vi "Test TS530A Remote Control.vi"() -> ()   [LabVIEW 2012]
doc: "Application example"
uses:
  <vilib>/Analysis/baseanly.llb/Mean (DBL).vi
  <vilib>/Analysis/NI_AALBase.lvlib
panel:
  out "SET POINT":u16
  out "MEASURED":dbl
  out "RESULTS":dbl[](array[numeric])
  in  "WHAT TO TEST":enum16{"PARAMS AND SET POINT", "ONLY SET POINT"}(ring)=enum."ONLY SET POINT"
  in  "VISA RESOURCE":refnum<visa-resource-name>="COM4"
  # "Test TS530A Remote Control.vi"
  # "NOTE: The 37-way data cable connecting the AVS-47B and TS-530A is needed for this test\n\nThis test VI goes through all PID parameters, turning on each of the TS-530A front panel\nstatus LEDs if the \"what to test\" control is \"params and set point\".  Then the VI \nproceeds to program the analog set point to values 2^n where n=0...14. The \"measured\" \nindicator shows the last result, while the \"results\" array is filled after the VI has run\nto the end. \n\nThe measured set point values may deviate from the ideal values by some hundred\nmicrovolts because of the finite accuracy of the D/A and A/D converters. \n    Operating range of the D/A converter starts from 1 and therefore the  very lowest \nreadings (<10..30) may be quite erroneous."
  # "1"
  # "2"
  # "4"
  # "8"
  # "16"
  # "32"
  # "64"
  # "128"
  # "256"
  # "512"
  # "1024"
  # "2048"
  # "4096"
  # "8192"
  # "16384"
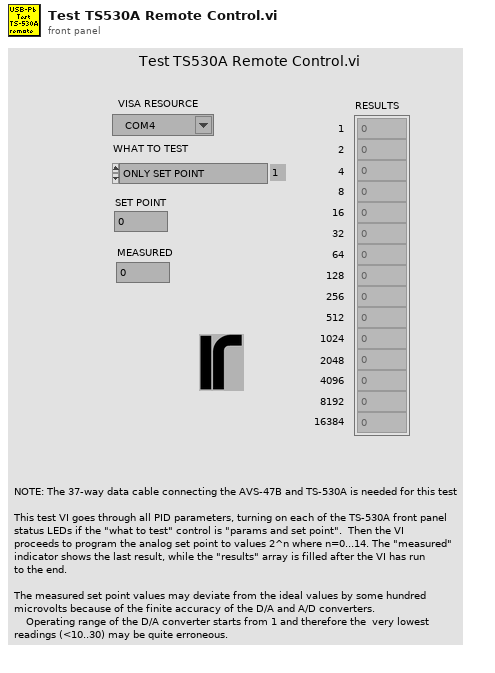
[diagram p1: front panel]
types:
  T1 = cluster{"VISA RESOURCE":refnum<visa-resource-name>, "PICOBUS ADDRESS":u8, "DISABLE AL":u8, "REMOTE":u8, "INPUT":u8, "CHANNEL":u8, "RANGE":u8, "EXCITATION":u8, "DISPLAY":u8, "DIGITAL REFERENCE":u16, "SET POINT":dbl, "PROP GAIN":u8, "INTG":u8, "DERIV":u8, "POWER BIAS":u8, "POWER RANGE":u8, "INFO STRING":string, "HEATER RESISTANCE":dbl, "INTERVAL":u8, " SENSOR dR/dT":u8}
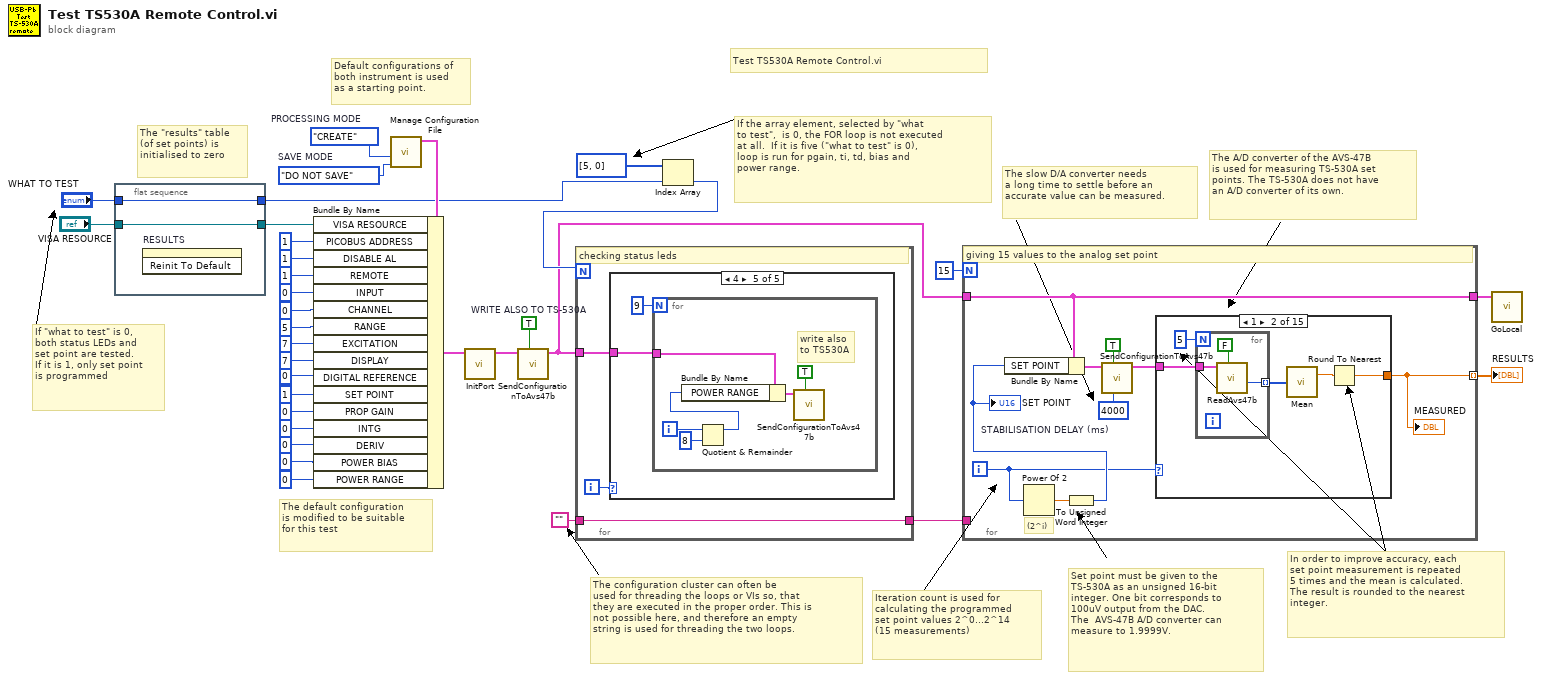
[diagram p0: block diagram]
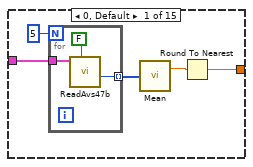
[diagram p2: hidden frame]
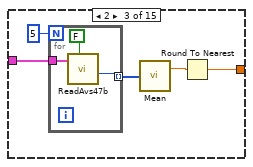
[diagram p3: hidden frame]
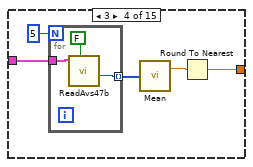
[diagram p4: hidden frame]
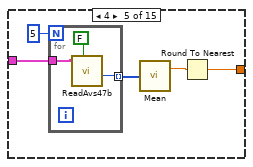
[diagram p5: hidden frame]
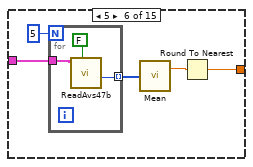
[diagram p6: hidden frame]
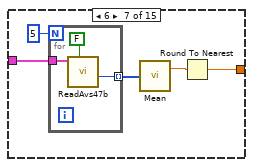
[diagram p7: hidden frame]
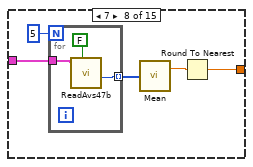
[diagram p8: hidden frame]
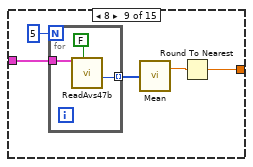
[diagram p9: hidden frame]
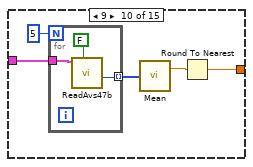
[diagram p10: hidden frame]
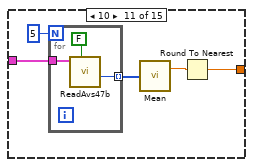
[diagram p11: hidden frame]
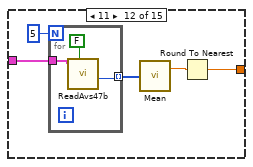
[diagram p12: hidden frame]
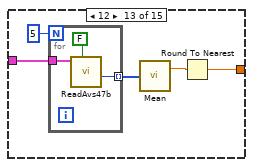
[diagram p13: hidden frame]
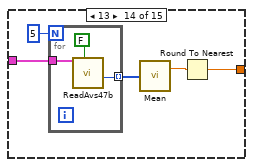
[diagram p14: hidden frame]
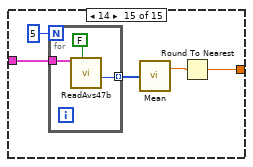
[diagram p15: hidden frame]
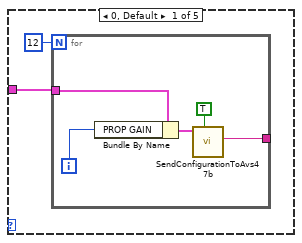
[diagram p16: hidden frame]
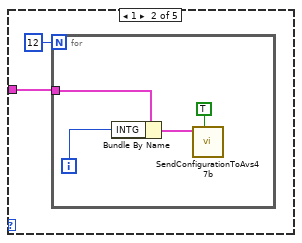
[diagram p17: hidden frame]
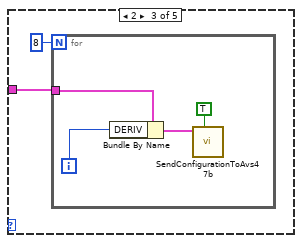
[diagram p18: hidden frame]
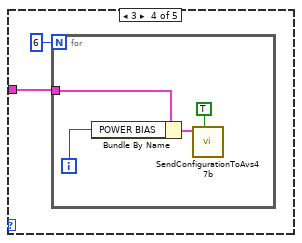
[diagram p19: hidden frame]
diagram:
  w3 = enum16{"DO NOT SAVE", "SAVE .CNF FILE"}."DO NOT SAVE"  # SAVE MODE
  w4 = enum16{"NONE", "READ", "CREATE"}."CREATE"  # PROCESSING MODE
  w17 = TRUE  # WRITE ALSO TO TS-530A
  # "Default configurations of \nboth instrument is used\nas a starting point."
  # "Test TS530A Remote Control.vi"
  # "The A/D converter of the AVS-47B\nis used for measuring TS-530A set\npoints. The TS-530A does not have\nan A/D converter of its own."
  # "If the array element, selected by \"what\nto test\",  is 0, the FOR loop is not executed \nat all.  If it is five (\"what to test\" is 0),\nloop is run for pgain, ti, td, bias and \npower range."
  # "The configuration cluster can often be\nused for threading the loops or VIs so, that \nthey are executed in the proper order. This is \nnot possible here, and therefore an empty \nstring is used for threading the two loops."
  # "Iteration count is used for\ncalculating the programmed\nset point values 2^0...2^14\n(15 measurements)"
  # "In order to improve accuracy, each \nset point measurement is repeated \n5 times and the mean is calculated. \nThe result is rounded to the nearest \ninteger."
  # "The slow D/A converter needs\na long time to settle before an\naccurate value can be measured."
  # "Set point must be given to the \nTS-530A as an unsigned 16-bit \ninteger. One bit corresponds to\n100uV output from the DAC. \nThe  AVS-47B A/D converter can \nmeasure to 1.9999V."
  # "If \"what to test\" is 0,\nboth status LEDs and \nset point are tested.\nIf it is 1, only set point\nis programmed"
  # "The default configuration\nis modified to be suitable\nfor this test"
  # "The \"results\" table\n(of set points) is \ninitialised to zero"
  n1 = flat-sequence {
    tunnel: "VISA RESOURCE" -> [w35]
    tunnel: [w35] -> w11
    tunnel: "WHAT TO TEST" -> [w34]
    tunnel: [w34] -> w9
    frame #0 {
      n2 = invoke on="RESULTS" class="Arr (strict)" method="Reinit To Default"() -> ()  [unwired: 3 in, 3 out]
    }
  }
  n3 = call "Manage Configuration File.vi"("SAVE MODE"=w3, "PROCESSING MODE"=w4) -> ("CONFIGURATION CLUSTER OUT"=w33:T1)  [unwired: 9 in]
  n4 = Bundle By Name(cluster=w33, "VISA RESOURCE"=w11, "PICOBUS ADDRESS"=u8 1, "DISABLE AL"=u8 1 ("PICOBUS ADDRESS"), "REMOTE"=u8 1 ("PICOBUS ADDRESS"), "INPUT"=u8 0 ("PICOBUS ADDRESS"), "CHANNEL"=u8 0 ("PICOBUS ADDRESS"), "RANGE"=u8 5 ("PICOBUS ADDRESS"), "EXCITATION"=u8 7 ("PICOBUS ADDRESS"), "DISPLAY"=u8 7 ("PICOBUS ADDRESS"), "DIGITAL REFERENCE"=u16 0, "SET POINT"=u16 1, "PROP GAIN"=u8 0 ("PICOBUS ADDRESS"), "INTG"=u8 0 ("PICOBUS ADDRESS"), "DERIV"=u8 0 ("PICOBUS ADDRESS"), "POWER BIAS"=u8 0 ("PICOBUS ADDRESS"), "POWER RANGE"=u8 0 ("PICOBUS ADDRESS")) -> (w2:T1)
  n5 = call "InitPort.vi"("CONFIGURATION CLUSTER"=w2) -> ("UNMODIFIED CONFIGURATION CLUSTER"=w1:T1)  [unwired: 6 in, 2 out]
  n6 = call "SendConfigurationToAvs47b.vi"("WRITE ALSO TO TS-530A"=w17, "CONFIGURATION CLUSTER"=w1) -> ("UNMODIFIED CONFIGURATION CLUSTER"=w7:T1)  [unwired: 6 in, 3 out]
  n7 = Index Array(array=i32[] [5, 0], index=w9) -> (element=w13:i32)
  n8 = for {
    N: w13 -> [_]
    tunnel: w7 -> [w37]
    tunnel: "" -> [w36]
    tunnel: [w36] -> w5
    i -> [w38]
    # "checking status leds"
    n9 = case shown="4" w38 {
      tunnel: w37 -> [w39 w46 w52 w58 w64]
      frame 0, Default {
        n10 = for {
          N: 12 -> [_]
          tunnel: w39 -> [w42]
          tunnel: [w41] -> _
          i -> [w45]
          n11 = Bundle By Name(cluster=w42, "PROP GAIN"=w45) -> (w44:T1)
          n12 = call "SendConfigurationToAvs47b.vi"("WRITE ALSO TO TS-530A"=TRUE, "CONFIGURATION CLUSTER"=w44) -> ("AVS47B TXSTR"=w41:string)  [unwired: 6 in, 3 out]
        }
      }
      frame 1 {
        n13 = for {
          N: 12 -> [_]
          tunnel: w46 -> [w48]
          i -> [w51]
          n14 = Bundle By Name(cluster=w48, "INTG"=w51) -> (w50:T1)
          n15 = call "SendConfigurationToAvs47b.vi"("WRITE ALSO TO TS-530A"=TRUE, "CONFIGURATION CLUSTER"=w50) -> ()  [unwired: 6 in, 4 out]
        }
      }
      frame 2 {
        n16 = for {
          N: 8 -> [_]
          tunnel: w52 -> [w54]
          i -> [w57]
          n17 = Bundle By Name(cluster=w54, "DERIV"=w57) -> (w56:T1)
          n18 = call "SendConfigurationToAvs47b.vi"("WRITE ALSO TO TS-530A"=TRUE, "CONFIGURATION CLUSTER"=w56) -> ()  [unwired: 6 in, 4 out]
        }
      }
      frame 3 {
        n19 = for {
          N: 6 -> [_]
          tunnel: w58 -> [w60]
          i -> [w63]
          n20 = Bundle By Name(cluster=w60, "POWER BIAS"=w63) -> (w62:T1)
          n21 = call "SendConfigurationToAvs47b.vi"("WRITE ALSO TO TS-530A"=TRUE, "CONFIGURATION CLUSTER"=w62) -> ()  [unwired: 6 in, 4 out]
        }
      }
      frame 4 {
        n22 = for {
          N: 9 -> [_]
          tunnel: w64 -> [w66]
          i -> [w69]
          # "write also \nto TS530A"
          n23 = Quotient & Remainder(x=w69, y=8) -> (x-y*floor(x/y)=w67:i32)  [unwired: 1 out]
          n24 = Bundle By Name(cluster=w66, "POWER RANGE"=w67) -> (w71:T1)
          n25 = call "SendConfigurationToAvs47b.vi"("WRITE ALSO TO TS-530A"=TRUE, "CONFIGURATION CLUSTER"=w71) -> ()  [unwired: 6 in, 4 out]
        }
      }
    }
  }
  n26 = for {
    N: 15 -> [_]
    tunnel: w7 -> [w73]
    tunnel: [w73] -> w15
    tunnel: [w72] -> w8 mode=indexing
    tunnel: w5 -> [_]
    i -> [w75]
    w76 = 4000  # STABILISATION DELAY (ms)
    # "(2^i)"
    # "giving 15 values to the analog set point"
    n27 = Power Of 2(x=w75) -> (2^x=w78:dbl)
    n28 = To Unsigned Word Integer(number=w78) -> (unsigned 16bit integer=w77:u16)
    "SET POINT" <- w77
    n29 = Bundle By Name(cluster=w73, "SET POINT"=w77) -> (w80:T1)
    n30 = call "SendConfigurationToAvs47b.vi"("STABILISATION DELAY (ms)"=w76, "WRITE ALSO TO TS-530A"=TRUE, "CONFIGURATION CLUSTER"=w80) -> ("UNMODIFIED CONFIGURATION CLUSTER"=w74:T1)  [unwired: 5 in, 3 out]
    n31 = case shown="1" w75 {
      tunnel: w74 -> [w85 w93 w101 w109 w117 w125 w133 w141 w149 w157 w165 w173 w181 w189 w197]
      tunnel: [w81 w89 w97 w105 w113 w121 w129 w137 w145 w153 w161 w169 w177 w185 w193] -> w72
      frame 0, Default {
        n32 = for {
          N: 5 -> [_]
          tunnel: w85 -> [w88]
          tunnel: [w87] -> w83 mode=indexing
          n33 = call "ReadAvs47b.vi"("SYNCHRONISE TO ADC"=FALSE ("SYNCHRONIZE TO ADC"), "CONFIGURATION CLUSTER"=w88) -> ("ADC"=w87:i32)  [unwired: 4 in, 5 out]
        }
        n34 = call-poly <vilib>:"Mean.vi"("X"=w83) -> ("mean"=w82:dbl)  [unwired: 1 out]
        n35 = Round To Nearest(number=w82) -> (nearest integer value=w81:dbl)
      }
      frame 1 {
        n36 = for {
          N: 5 -> [_]
          tunnel: w93 -> [w96]
          tunnel: [w95] -> w91 mode=indexing
          n37 = call "ReadAvs47b.vi"("SYNCHRONISE TO ADC"=FALSE ("SYNCHRONIZE TO ADC"), "CONFIGURATION CLUSTER"=w96) -> ("ADC"=w95:i32)  [unwired: 4 in, 5 out]
        }
        n38 = call-poly <vilib>:"Mean.vi"("X"=w91) -> ("mean"=w90:dbl)  [unwired: 1 out]
        n39 = Round To Nearest(number=w90) -> (nearest integer value=w89:dbl)
      }
      frame 2 {
        n40 = for {
          N: 5 -> [_]
          tunnel: w101 -> [w103]
          tunnel: [w102] -> w99 mode=indexing
          n41 = call "ReadAvs47b.vi"("SYNCHRONISE TO ADC"=FALSE ("SYNCHRONIZE TO ADC"), "CONFIGURATION CLUSTER"=w103) -> ("ADC"=w102:i32)  [unwired: 4 in, 5 out]
        }
        n42 = call-poly <vilib>:"Mean.vi"("X"=w99) -> ("mean"=w98:dbl)  [unwired: 1 out]
        n43 = Round To Nearest(number=w98) -> (nearest integer value=w97:dbl)
      }
      frame 3 {
        n44 = for {
          N: 5 -> [_]
          tunnel: w109 -> [w111]
          tunnel: [w110] -> w107 mode=indexing
          n45 = call "ReadAvs47b.vi"("SYNCHRONISE TO ADC"=FALSE ("SYNCHRONIZE TO ADC"), "CONFIGURATION CLUSTER"=w111) -> ("ADC"=w110:i32)  [unwired: 4 in, 5 out]
        }
        n46 = call-poly <vilib>:"Mean.vi"("X"=w107) -> ("mean"=w106:dbl)  [unwired: 1 out]
        n47 = Round To Nearest(number=w106) -> (nearest integer value=w105:dbl)
      }
      frame 4 {
        n48 = for {
          N: 5 -> [_]
          tunnel: w117 -> [w119]
          tunnel: [w118] -> w115 mode=indexing
          n49 = call "ReadAvs47b.vi"("SYNCHRONISE TO ADC"=FALSE ("SYNCHRONIZE TO ADC"), "CONFIGURATION CLUSTER"=w119) -> ("ADC"=w118:i32)  [unwired: 4 in, 5 out]
        }
        n50 = call-poly <vilib>:"Mean.vi"("X"=w115) -> ("mean"=w114:dbl)  [unwired: 1 out]
        n51 = Round To Nearest(number=w114) -> (nearest integer value=w113:dbl)
      }
      frame 5 {
        n52 = for {
          N: 5 -> [_]
          tunnel: w125 -> [w127]
          tunnel: [w126] -> w123 mode=indexing
          n53 = call "ReadAvs47b.vi"("SYNCHRONISE TO ADC"=FALSE ("SYNCHRONIZE TO ADC"), "CONFIGURATION CLUSTER"=w127) -> ("ADC"=w126:i32)  [unwired: 4 in, 5 out]
        }
        n54 = call-poly <vilib>:"Mean.vi"("X"=w123) -> ("mean"=w122:dbl)  [unwired: 1 out]
        n55 = Round To Nearest(number=w122) -> (nearest integer value=w121:dbl)
      }
      frame 6 {
        n56 = for {
          N: 5 -> [_]
          tunnel: w133 -> [w135]
          tunnel: [w134] -> w131 mode=indexing
          n57 = call "ReadAvs47b.vi"("SYNCHRONISE TO ADC"=FALSE ("SYNCHRONIZE TO ADC"), "CONFIGURATION CLUSTER"=w135) -> ("ADC"=w134:i32)  [unwired: 4 in, 5 out]
        }
        n58 = call-poly <vilib>:"Mean.vi"("X"=w131) -> ("mean"=w130:dbl)  [unwired: 1 out]
        n59 = Round To Nearest(number=w130) -> (nearest integer value=w129:dbl)
      }
      frame 7 {
        n60 = for {
          N: 5 -> [_]
          tunnel: w141 -> [w143]
          tunnel: [w142] -> w139 mode=indexing
          n61 = call "ReadAvs47b.vi"("SYNCHRONISE TO ADC"=FALSE ("SYNCHRONIZE TO ADC"), "CONFIGURATION CLUSTER"=w143) -> ("ADC"=w142:i32)  [unwired: 4 in, 5 out]
        }
        n62 = call-poly <vilib>:"Mean.vi"("X"=w139) -> ("mean"=w138:dbl)  [unwired: 1 out]
        n63 = Round To Nearest(number=w138) -> (nearest integer value=w137:dbl)
      }
      frame 8 {
        n64 = for {
          N: 5 -> [_]
          tunnel: w149 -> [w151]
          tunnel: [w150] -> w147 mode=indexing
          n65 = call "ReadAvs47b.vi"("SYNCHRONISE TO ADC"=FALSE ("SYNCHRONIZE TO ADC"), "CONFIGURATION CLUSTER"=w151) -> ("ADC"=w150:i32)  [unwired: 4 in, 5 out]
        }
        n66 = call-poly <vilib>:"Mean.vi"("X"=w147) -> ("mean"=w146:dbl)  [unwired: 1 out]
        n67 = Round To Nearest(number=w146) -> (nearest integer value=w145:dbl)
      }
      frame 9 {
        n68 = for {
          N: 5 -> [_]
          tunnel: w157 -> [w159]
          tunnel: [w158] -> w155 mode=indexing
          n69 = call "ReadAvs47b.vi"("SYNCHRONISE TO ADC"=FALSE ("SYNCHRONIZE TO ADC"), "CONFIGURATION CLUSTER"=w159) -> ("ADC"=w158:i32)  [unwired: 4 in, 5 out]
        }
        n70 = call-poly <vilib>:"Mean.vi"("X"=w155) -> ("mean"=w154:dbl)  [unwired: 1 out]
        n71 = Round To Nearest(number=w154) -> (nearest integer value=w153:dbl)
      }
      frame 10 {
        n72 = for {
          N: 5 -> [_]
          tunnel: w165 -> [w167]
          tunnel: [w166] -> w163 mode=indexing
          n73 = call "ReadAvs47b.vi"("SYNCHRONISE TO ADC"=FALSE ("SYNCHRONIZE TO ADC"), "CONFIGURATION CLUSTER"=w167) -> ("ADC"=w166:i32)  [unwired: 4 in, 5 out]
        }
        n74 = call-poly <vilib>:"Mean.vi"("X"=w163) -> ("mean"=w162:dbl)  [unwired: 1 out]
        n75 = Round To Nearest(number=w162) -> (nearest integer value=w161:dbl)
      }
      frame 11 {
        n76 = for {
          N: 5 -> [_]
          tunnel: w173 -> [w175]
          tunnel: [w174] -> w171 mode=indexing
          n77 = call "ReadAvs47b.vi"("SYNCHRONISE TO ADC"=FALSE ("SYNCHRONIZE TO ADC"), "CONFIGURATION CLUSTER"=w175) -> ("ADC"=w174:i32)  [unwired: 4 in, 5 out]
        }
        n78 = call-poly <vilib>:"Mean.vi"("X"=w171) -> ("mean"=w170:dbl)  [unwired: 1 out]
        n79 = Round To Nearest(number=w170) -> (nearest integer value=w169:dbl)
      }
      frame 12 {
        n80 = for {
          N: 5 -> [_]
          tunnel: w181 -> [w183]
          tunnel: [w182] -> w179 mode=indexing
          n81 = call "ReadAvs47b.vi"("SYNCHRONISE TO ADC"=FALSE ("SYNCHRONIZE TO ADC"), "CONFIGURATION CLUSTER"=w183) -> ("ADC"=w182:i32)  [unwired: 4 in, 5 out]
        }
        n82 = call-poly <vilib>:"Mean.vi"("X"=w179) -> ("mean"=w178:dbl)  [unwired: 1 out]
        n83 = Round To Nearest(number=w178) -> (nearest integer value=w177:dbl)
      }
      frame 13 {
        n84 = for {
          N: 5 -> [_]
          tunnel: w189 -> [w191]
          tunnel: [w190] -> w187 mode=indexing
          n85 = call "ReadAvs47b.vi"("SYNCHRONISE TO ADC"=FALSE ("SYNCHRONIZE TO ADC"), "CONFIGURATION CLUSTER"=w191) -> ("ADC"=w190:i32)  [unwired: 4 in, 5 out]
        }
        n86 = call-poly <vilib>:"Mean.vi"("X"=w187) -> ("mean"=w186:dbl)  [unwired: 1 out]
        n87 = Round To Nearest(number=w186) -> (nearest integer value=w185:dbl)
      }
      frame 14 {
        n88 = for {
          N: 5 -> [_]
          tunnel: w197 -> [w199]
          tunnel: [w198] -> w195 mode=indexing
          n89 = call "ReadAvs47b.vi"("SYNCHRONISE TO ADC"=FALSE ("SYNCHRONIZE TO ADC"), "CONFIGURATION CLUSTER"=w199) -> ("ADC"=w198:i32)  [unwired: 4 in, 5 out]
        }
        n90 = call-poly <vilib>:"Mean.vi"("X"=w195) -> ("mean"=w194:dbl)  [unwired: 1 out]
        n91 = Round To Nearest(number=w194) -> (nearest integer value=w193:dbl)
      }
    }
    "MEASURED" <- w72
  }
  "RESULTS" <- w8
  n92 = call "GoLocal.vi"("CONFIGURATION CLUSTER"=w15) -> ()  [unwired: 10 in, 1 out]
